vi "Nicholas IO Server.vi"() -> ()   [LabVIEW 2016]
uses:
  RS485 In.ctl
  Serial Data In.ctl
  <vilib>/rvi/eio/common/nirviEmuClasses.ctl
  <vilib>/Platform/TimedLoop/XDataNode/timing_clust.ctl
  <vilib>/Platform/TimedLoop/XDataNode/nitl_modes.ctl
  <vilib>/Platform/TimedLoop/XDataNode/wakeup.ctl
  <vilib>/rvi/FXPMathLib/basic elements/FxpIntAccumulator/subVIs/nifxpmath_IntAccumulator_SimConfig.ctl
  <vilib>/rvi/Emulation/niFpgaSctlEmulationGetInTimedLoop.vi
  <vilib>/rvi/Emulation/niFpgaProcessEmulError.vi
  <vilib>/rvi/eio/common/nirviEmuTemplateMethod_errors.vi
  <vilib>/rvi/Emulation/niFpgaEmulationIsFPGAContextNoSignature.vi
  <vilib>/rvi/DataTransferAndStorage/Container/Common/niFpgaContainerGetUniqueNameForEmu.vi
  <vilib>/rvi/Memory/Memory_Emulation/niFpgaMemoryEmulationCacheClearOnFirstRun.vi
  <vilib>/rvi/Memory/Memory_Emulation/nirvimemoryEmulationManagerCache_MakeExclusive.vi
  <vilib>/rvi/Memory/Memory_Emulation/niFpgaMemoryEmulationValidateCache.vi
  <vilib>/rvi/Memory/Memory_Emulation/nirvimemoryEmulationManagerCache_InsertValue.vi
  <vilib>/Utility/error.llb/Clear Errors.vi
  <vilib>/rvi/Memory/Memory_Emulation/nirvimemoryEmulationManagerCache_ReleaseExclusive.vi
  <vilib>/rvi/Memory/Memory_Emulation/nirvimemoryEmulationManagerCache_GetValue.vi
  <vilib>/rvi/Memory/Memory_Emulation/nirvimemoryEmulationManagerCache_SetValue.vi
  <vilib>/rvi/Emulation/niFpgaGetClockAttributes.vi
  <vilib>/rvi/Emulation/niFpgaEmulationReportErrorSimple.vi
  <vilib>/rvi/Emulation/niFpgaCriticalErrorInLSC.vi
  <vilib>/rvi/FXPMathLib/basic elements/FxpIntAccumulator/simVIs/DllFxpIntAccumulator_sub.vi
  <vilib>/eio/EIOGrowableMethodNode/genericMethod/EIOGrowableMethodNode.xnode
  <vilib>/rvi/eio/nirviEIOMethodImplementation/nirviEIOMethodImplementation.xnode
  <vilib>/rvi/eio/nirviErrorMerge/nirviErrorMerge.xnode
  <vilib>/rvi/DataTransferAndStorage/Container/XNode/niFpgaContainer.xnode
  <vilib>/rvi/DataTransferAndStorage/Register/Emulation/niFpgaRegisterEmulation.vi
  <vilib>/Platform/TimedLoop/XDataNode/XDataNode.xnode
  <vilib>/eio/EIONode/EIONode.xnode
  <vilib>/rvi/FXPMathLib/basic elements/FxpIntAccumulator/XNode/nifxpmath_IntAccumulator.xnode
  <vilib>/rvi/FXPMathLib/basic elements/FxpDiscreteDelay/XNode/nifxpmath_DiscreteDelay.xnode
  <vilib>/rvi/FXPMathLib/FxpMul/XNode/nifxpmath_Multiplier.xnode
  <vilib>/Platform/TimedLoop/XDataNode/XDNodeRunTimeDep.lvlib
  <vilib>/rvi/FXPMathLib/sim/FxpSim.dll
  Port.ctl
panel:
  in  "f0":fxp<+,32,0>
  out "DI Out":u8
  out "DO Out":u16
  in  "DO In":u16
  out "Version":i64=3288624
  in  "pDC":fxp<+,32,0>
  out "Port4 Out":T1
  in  "Port4 In":T2={"Data"=[0, 0, 0, 0, 0, 0, 0, 0, 0, 0, 0, 0, 0, 0, 0, 0, 0, 0, 0, 0], "NumBytes"=0, "RS485_Cmd"=enum."Idle", "Timeout (ms)"=0}
  out "Port3 Out":T1
  in  "Port3 In":T2={"Data"=[0, 0, 0, 0, 0, 0, 0, 0, 0, 0, 0, 0, 0, 0, 0, 0, 0, 0, 0, 0], "NumBytes"=0, "RS485_Cmd"=enum."Idle", "Timeout (ms)"=0}
  out "Port2 Out":T1
  in  "Port2 In":T2={"Data"=[0, 0, 0, 0, 0, 0, 0, 0, 0, 0, 0, 0, 0, 0, 0, 0, 0, 0, 0, 0], "NumBytes"=0, "RS485_Cmd"=enum."Idle", "Timeout (ms)"=0}
  in  "Port1 In":T2={"Data"=[0, 0, 0, 0, 0, 0, 0, 0, 0, 0, 0, 0, 0, 0, 0, 0, 0, 0, 0, 0], "NumBytes"=0, "RS485_Cmd"=enum."Idle", "Timeout (ms)"=0}
  out "Port1 Out":T1
  in  "Transmit?":bool
  in  "CRDSampData":u32
  in  "Speaker":cluster{"Vscale":fxp<+,32,0>, "Offset":i16}
  in  "Stop":bool
  out "HK Data":fxp<+/-,16,5>[](array[numeric])
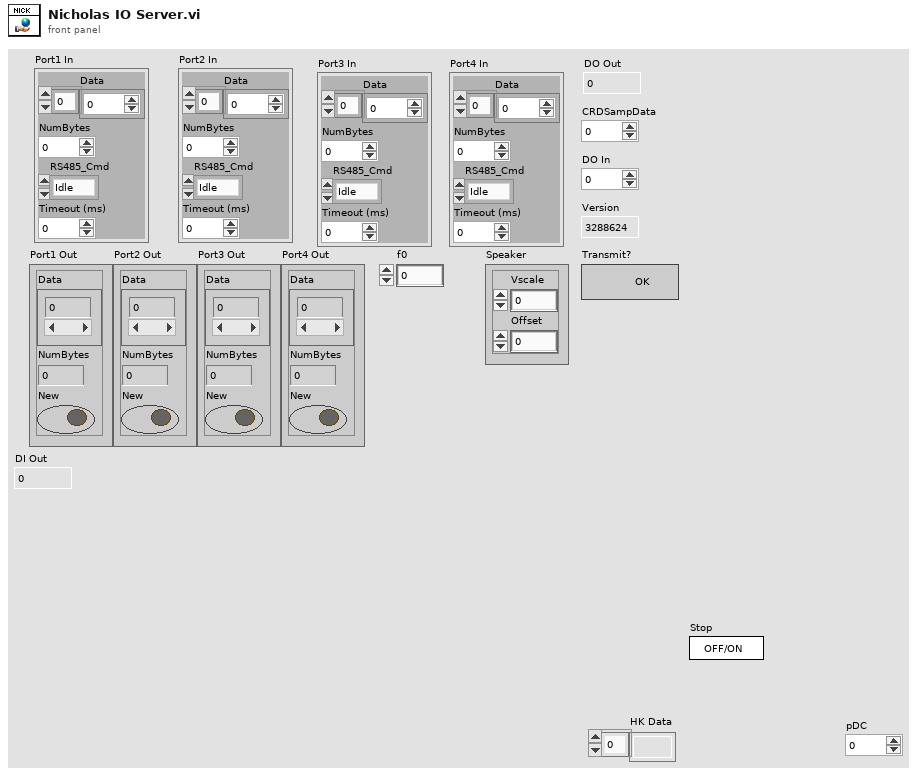
[diagram p1: front panel]
types:
  T1 = typedef "RS485 In.ctl" = cluster{"Data":u8[], "NumBytes":i32, "New":bool}
  T2 = typedef "Serial Data In.ctl" = cluster{"Data":u8[], "NumBytes":i32, "RS485_Cmd":enum8{"Read", "Write", "Idle"}, "Timeout (ms)":i32}
  T3 = typedef "nirviEmuClasses.ctl" = enum16{"IO Read", "IO Write", "Method", "Property Read", "Property Write"}
  T4 = typedef "Port.ctl" = enum8{"Port 1", "Port 2", "Port 3", "Port 4", "None"}
  T5 = typedef "XDNodeRunTimeDep.lvlib/timing_clust.ctl" = cluster{"Expected End [f-1]":u64, "Actual End [f-1]":u64, "Finished Late? [f-1]":bool, "Expected End [i-1]":u64, "Actual End [i-1]":u64, "Finished Late? [i-1]":bool, "Expected Start [i]":u64, "Actual Start [i]":u64, "Expected Start [f]":u64, "Actual Start [f]":u64, "Source Name":string, "Structure Name":string, "Period":i64, "Deadline":i64, "Offset":i64, "Start":i64, "Priority":i32, "Timeout":i32, "Mode":T6, "Wakeup Reason":T7, "Error":errorcluster, "Source Type":string, "Secondary Source Type":string, "Global End Time":u64, "Global Start Time":u64, "Frame Duration":u64, "Iteration Duration":u64, "Assigned CPU":i32, "I/O Scan Engine Mode":u32}
  T6 = typedef "XDNodeRunTimeDep.lvlib/nitl_modes.ctl" = enum32{"No Change", "Process missed periods, maintain original phase", "Discard missed periods, maintain original phase", "Process missed periods, ignore original phase", "Discard missed periods, ignore original phase"}
  T7 = typedef "XDNodeRunTimeDep.lvlib/wakeup.ctl" = enum32{"Normal", "Aborted", "Asynchronous wakeup", "Timing source error", "Timed loop error", "Timeout"}
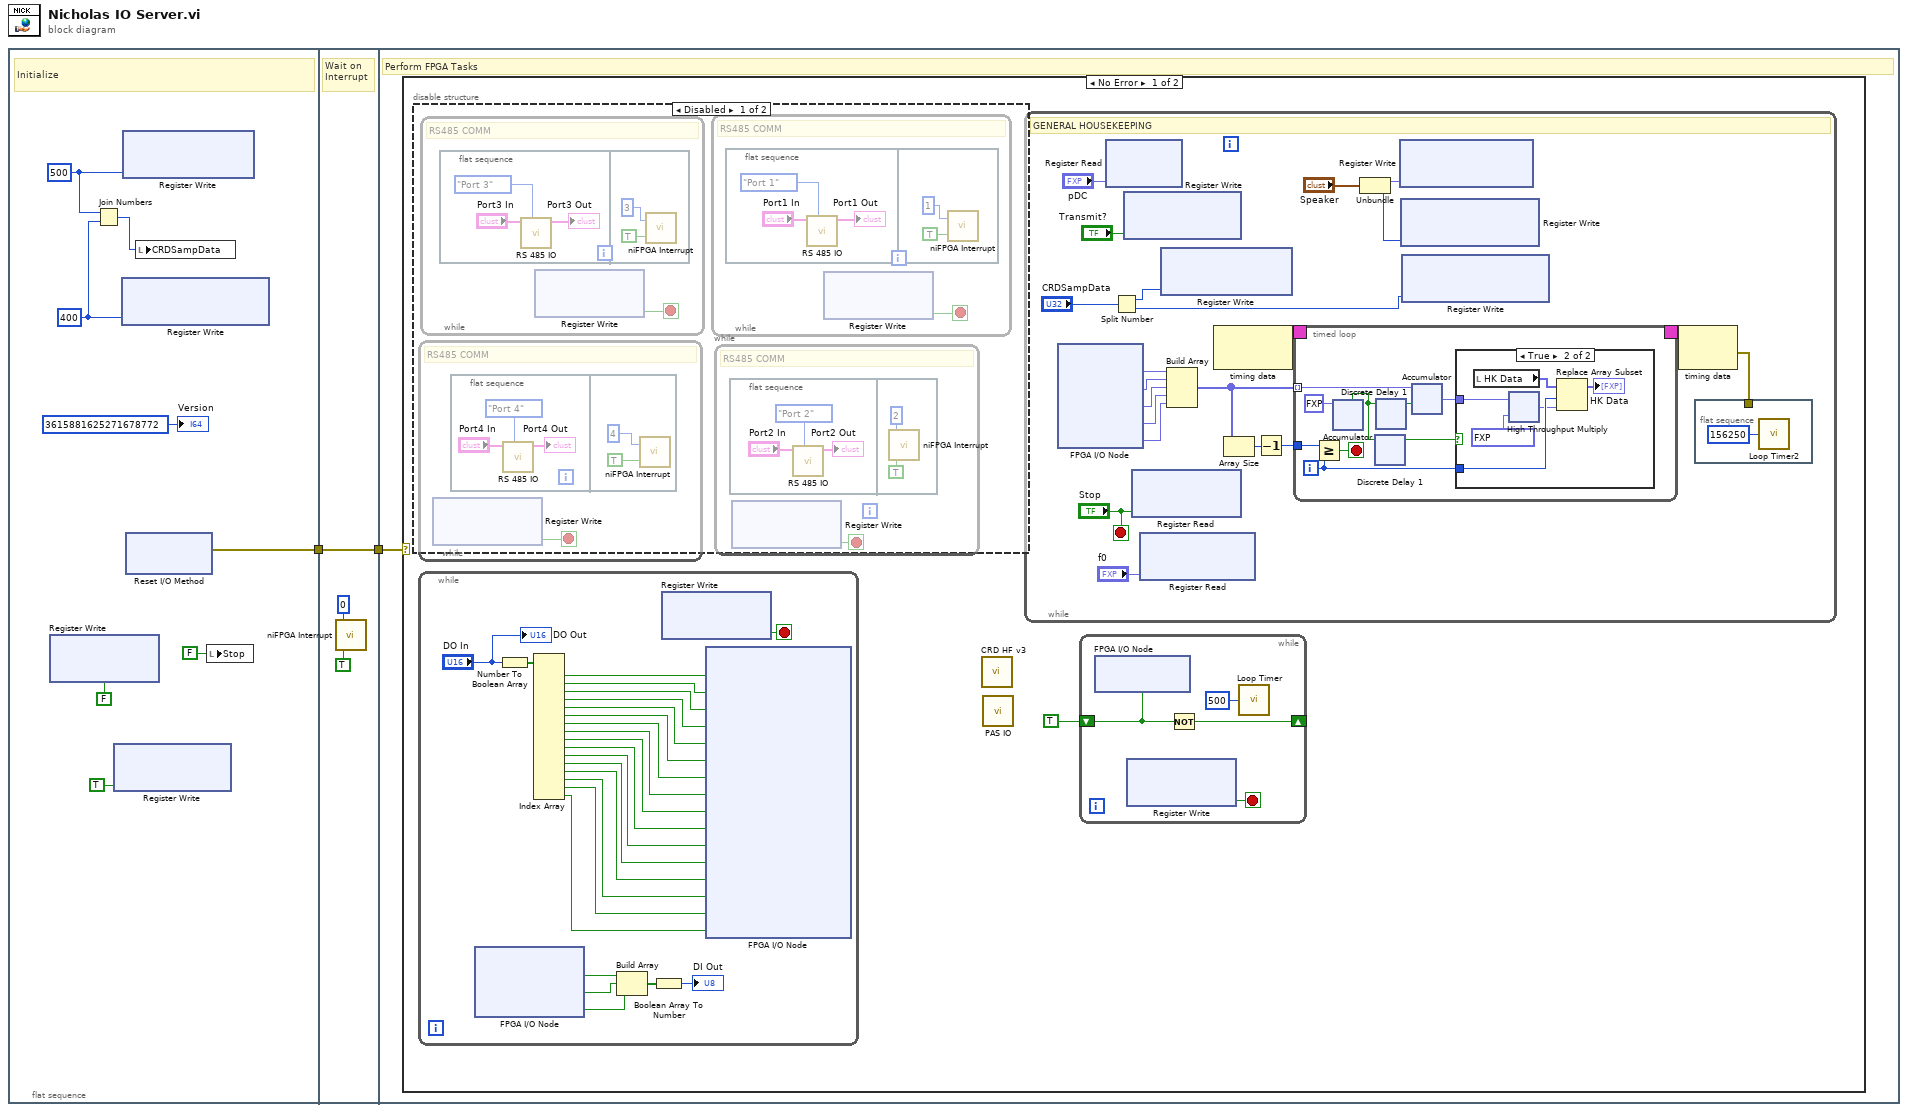
[diagram p0: block diagram]
diagram:
  n1 = flat-sequence {
    tunnel: [w10] -> w2
    tunnel: w2 -> [w57]
    tunnel: [w57] -> w1
    tunnel: w1 -> [w58]
    frame #0 {
      w5 = u16 500 ("Data")
      w4 = u16 400 ("Data")
      # "Initialize"
      n2 = xnode ("Register Write")("Data"=FALSE) -> ()  [unwired: 1 in, 1 out]
      n3 = Join Numbers(hi=w5, lo=w4) -> ((hi.lo)=w3:u32)
      n4 = xnode ("Register Write")("Data"=TRUE) -> ()  [unwired: 1 in, 1 out]
      n5 = xnode ("Register Write")("Data"=w4) -> ()  [unwired: 1 in, 1 out]
      n6 = xnode ("Register Write")("Data"=w5) -> ()  [unwired: 1 in, 1 out]
      n7 = xnode "Reset I/O Method"() -> ("error out"=w10:errorcluster)  [unwired: 2 in, 1 out]
      n8 = local write "CRDSampData"(w3) -> ()
      n9 = local write "Stop"(FALSE ("Stop")) -> ()
      "Version" <- i64 3615881625271678772 ("Data")
    }
    frame #1 {
      # "Wait on Interrupt"
      n10 = call <vilib>:"niFPGA Interrupt.vi"("Wait Until Cleared (F)"=TRUE ("Wait Until Cleared"), "IRQ Number (0)"=u8 0 ("IRQ Number")) -> ()  [unwired: 1 in]
    }
    frame #2 {
      # "Perform FPGA Tasks"
      n11 = case shown="No Error" w58 {
        frame No Error {
          n12 = disable-structure shown="Disabled" {
            frame Disabled {
              n13 = while {
                stop <- w78 stop-if-true
                # "RS485 COMM"
                n14 = xnode ("Register Write")() -> ("Data"=w78:bool)  [unwired: 1 in, 1 out]
                n15 = flat-sequence {
                  frame #0 {
                    n16 = call "RS 485 IO.vi"("Port"=Port."Port 4", "Input in"="Port4 In") -> ("Input out"=→"Port4 Out":T1)  [unwired: 8 in]
                  }
                  frame #1 {
                    n17 = call <vilib>:"niFPGA Interrupt.vi"("Wait Until Cleared (F)"=TRUE, "IRQ Number (0)"=u8 4) -> ()  [unwired: 1 in]
                  }
                }
              }
              n18 = while {
                stop <- w60 stop-if-true
                # "RS485 COMM"
                n19 = flat-sequence {
                  frame #0 {
                    n20 = call "RS 485 IO.vi"("Port"=Port."Port 3", "Input in"="Port3 In") -> ("Input out"=→"Port3 Out":T1)  [unwired: 8 in]
                  }
                  frame #1 {
                    n21 = call <vilib>:"niFPGA Interrupt.vi"("Wait Until Cleared (F)"=TRUE, "IRQ Number (0)"=u8 3) -> ()  [unwired: 1 in]
                  }
                }
                n22 = xnode ("Register Write")() -> ("Data"=w60:bool)  [unwired: 1 in, 1 out]
              }
              n23 = while {
                stop <- w66 stop-if-true
                # "RS485 COMM"
                n24 = flat-sequence {
                  frame #0 {
                    n25 = call "RS 485 IO.vi"("Port"=Port."Port 1", "Input in"="Port1 In") -> ("Input out"=→"Port1 Out":T1)  [unwired: 8 in]
                  }
                  frame #1 {
                    n26 = call <vilib>:"niFPGA Interrupt.vi"("Wait Until Cleared (F)"=TRUE, "IRQ Number (0)"=u8 1) -> ()  [unwired: 1 in]
                  }
                }
                n27 = xnode ("Register Write")() -> ("Data"=w66:bool)  [unwired: 1 in, 1 out]
              }
              n28 = while {
                stop <- w72 stop-if-true
                # "RS485 COMM"
                n29 = flat-sequence {
                  frame #0 {
                    n30 = call "RS 485 IO.vi"("Port"=Port."Port 2", "Input in"="Port2 In") -> ("Input out"=→"Port2 Out":T1)  [unwired: 8 in]
                  }
                  frame #1 {
                    n31 = call <vilib>:"niFPGA Interrupt.vi"("Wait Until Cleared (F)"=TRUE, "IRQ Number (0)"=u8 2) -> ()  [unwired: 1 in]
                  }
                }
                n32 = xnode ("Register Write")() -> ("Data"=w72:bool)  [unwired: 1 in, 1 out]
              }
            }
            frame Enabled {
            }
          }
          n33 = while {
            stop <- w111 stop-if-true
            n34 = xnode "FPGA I/O Node"() -> ("hb 1 status 1"=w92:bool, "hb 1 status 2"=w91:bool, "Interlock"=w90:bool)  [unwired: 3 in, 3 out]
            n35 = Number To Boolean Array(number="DO In") -> (Boolean array=w109:bool[])
            n36 = Index Array(array=w109) -> (element #1=w108:bool, element #2=w107:bool, element #3=w106:bool, element #4=w105:bool, element #5=w104:bool, element #6=w103:bool, element #7=w102:bool, element #8=w101:bool, element #9=w100:bool, element #10=w99:bool, element #11=w98:bool, element #12=w97:bool, element #13=w96:bool, element #14=w95:bool, element #15=w94:bool, element #16=w93:bool)  [unwired: 16 in]
            n37 = Build Array(w92, w91, w90) -> (w89:bool[])
            n38 = Boolean Array To Number(Boolean array=w89) -> (number=→"DI Out":u8)
            n39 = xnode ("Register Write")() -> ("Data"=w111:bool)  [unwired: 1 in, 1 out]
            n40 = xnode "FPGA I/O Node"("uv light ctl 1"=w108, "uv light ctl 2"=w107, "uv light enable"=w106, "Laser Enable"=w105, "PAS Speaker"=w104, "Compressor Enable"=w103, "Vacuum Pump"=w102, "O3 Add"=w101, "Scrubber Test"=w100, "Pressure Meas 1"=w99, "Pressure Meas 2"=w98, "hb 1 ctl 1"=w97, "hb 1 ctl 2"=w96, "CRD Laser Enable"=w95, "PMT Enable"=w94, "Fan Enable"=w93) -> ()  [unwired: 16 in, 16 out]
            "DO Out" <- "DO In"
          }
          n41 = call "CRD HF v3.vi"() -> ()  [unwired: 12 in]
          n42 = call "PAS IO.vi"() -> ()  [unwired: 20 in]
          n43 = while {
            stop <- "Stop" stop-if-true
            # "GENERAL HOUSEKEEPING"
            n44 = xnode "FPGA I/O Node"() -> ("Tcomp"=w126:fxp<+/-,26,5>, "TEC hot"=w127:fxp<+/-,26,5>, "Troom"=w128:fxp<+/-,26,5>, "Box"=w129:fxp<+/-,26,5>, "Cell"=w130:fxp<+/-,26,5>)  [unwired: 5 in, 5 out]
            n45 = xnode ("Register Read")("Data"="pDC") -> ()  [unwired: 1 in, 1 out]
            n46 = Split Number(x="CRDSampData") -> (hi(x)=w114:u16, lo(x)=w113:u16)
            n47 = xnode ("Register Write")("Data"="Transmit?") -> ()  [unwired: 1 in, 1 out]
            n48 = xnode ("Register Read")("Data"="Stop") -> ()  [unwired: 1 in, 1 out]
            n49 = xnode ("Register Read")("Data"="f0") -> ()  [unwired: 1 in, 1 out]
            n50 = xnode ("Register Write")("Data"=w114) -> ()  [unwired: 1 in, 1 out]
            n51 = Build Array(w126, w127, w128, w129, w130) -> (w125:fxp<+/-,26,5>[])
            n52 = node-c288() -> (w132:T5)  [unwired: 1 in]
            n53 = Array Size(array=w125) -> (size(s)=w124:i32)
            n54 = Decrement(x=w124) -> (x-1=w123:i32)
            n55 = timed-loop {
              timing: w132 -> [_]
              timing-out: [_] -> w131
              tunnel: w125 -> [w140] mode=indexing
              tunnel: w123 -> [w142]
              i -> [w134]
              stop <- w141 stop-if-true
              n56 = Greater Or Equal?(x=w142, y=w134) -> (x >= y?=w141:bool)
              n57 = xnode "Accumulator"("x"=fxp<+,1,1> 1.0) -> ("carry-out/inverted borrow-out"=w137:bool)  [unwired: 4 in, 1 out]
              n58 = xnode ("Discrete Delay 1")("D"=w137) -> ("Q"=w136:bool)
              n59 = xnode ("Discrete Delay 1")("D"=w137) -> ("Q"=w138:bool)
              n60 = xnode "Accumulator"("x"=w140, "load (F)"=w138) -> ("s"=w135:fxp<+/-,32,11>)  [unwired: 3 in, 1 out]
              n61 = case shown="True" w136 {
                tunnel: w135 -> [_ w148]
                tunnel: w134 -> [_ w146]
                frame False {
                }
                frame True {
                  n62 = local read "HK Data"() -> (w147:fxp<+/-,16,5>[])
                  n63 = xnode ("High Throughput Multiply")("x"=w148, "y"=fxp<+,32,1> 0.00390625) -> ("x*y"=w145:fxp<+/-,16,5>)
                  n64 = Replace Array Subset(array=w147, new element=w145, index=w146) -> (→"HK Data":fxp<+/-,16,5>[])
                }
              }
            }
            n65 = Unbundle("Speaker") -> ("Vscale"=w116:fxp<+,32,0>, "Offset"=w118:i16)
            n66 = xnode ("Register Write")("Data"=w116) -> ()  [unwired: 1 in, 1 out]
            n67 = xnode ("Register Write")("Data"=w118) -> ()  [unwired: 1 in, 1 out]
            n68 = xnode ("Register Write")("Data"=w113) -> ()  [unwired: 1 in, 1 out]
            n69 = node-c288(w131) -> (w122:errorcluster)
            n70 = flat-sequence {
              tunnel: w122 -> [_]
              frame #0 {
                n71 = call "Loop Timer2"("Count(Ticks)"=u32 156250 ("Count(mSec)")) -> ()  [unwired: 1 out]
              }
            }
          }
          n72 = while {
            shift-right: [w85] -> _
            shift-left: TRUE -> [w86]
            stop <- w84 stop-if-true
            n73 = xnode "FPGA I/O Node"("Heartbeat"=w86) -> ()  [unwired: 1 in, 1 out]
            n74 = xnode ("Register Write")() -> ("Data"=w84:bool)  [unwired: 1 in, 1 out]
            n75 = Not(x=w86) -> (.not. x?=w85:bool)
            n76 = call "Loop Timer"("Count(mSec)"=u32 500 ("Count(Ticks)")) -> ()  [unwired: 1 out]
          }
        }
        frame Error {
        }
      }
    }
  }
